vi "TestPanel.vi"() -> ()   [LabVIEW 2018]
uses:
  <vilib>/DAQmx/read.llb/DAQmx Read (Analog 1D Wfm NChan NSamp).vi
  <vilib>/DAQmx/create/channels.llb/DAQmx Create Channel (AI-Voltage-Basic).vi
  <vilib>/DAQmx/configure/timing.llb/DAQmx Timing (Sample Clock).vi
  <vilib>/DAQmx/miscellaneous.llb/DAQmx Fill In Error Info.vi
  <vilib>/measure/madcrms.llb/Basic Averaged DC-RMS for N Chan.vi
  <vilib>/measure/NI_MAPro.lvlib
panel:
  out "Voltage Chart":waveform(dbl)[](graph)
  out "Table Control":string[][](table)
  in  "Stop":bool
  in  "Manual Zero":bool
  # "Test Panel v1.0"
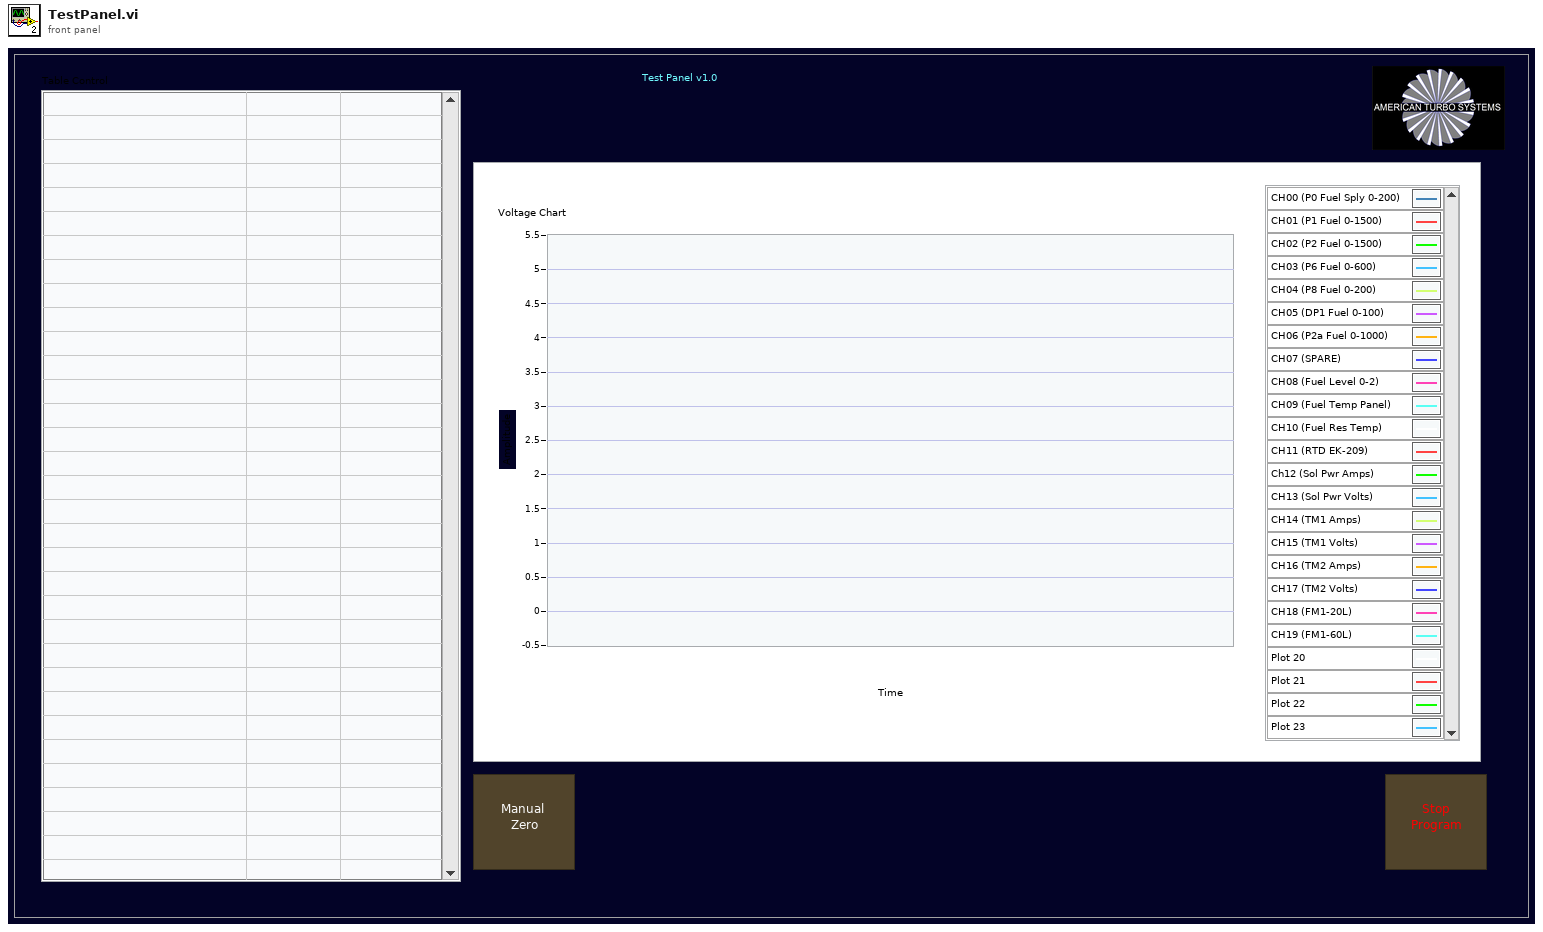
[diagram p1: front panel]
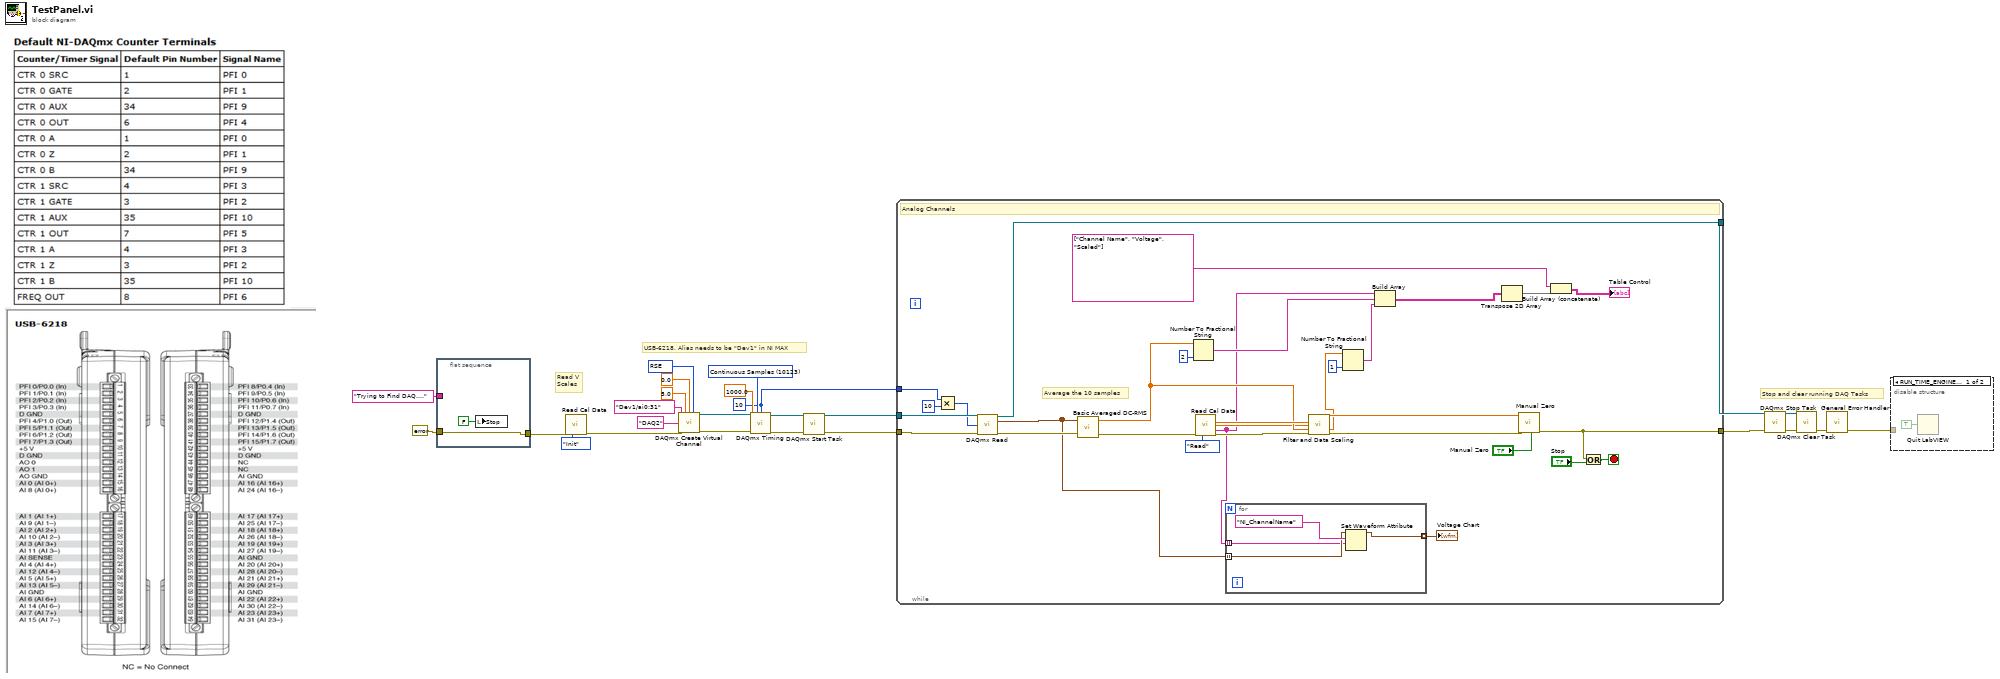
[diagram p0: block diagram]
diagram:
  w4 = 10 ("samples per channel")
  w21 = 10123 items=["Finite Samples"=10178, "Continuous Samples"=10123, "Hardware Timed Single Point"=12522] ("sample mode")
  w18 = 10083 items=["Default"=-1, "RSE"=10083, "NRSE"=10078, "Differential"=10106, "Pseudodifferential"=12529] ("input terminal configuration")
  # "USB-6218. Alias needs to be \"Dev1\" in NI MAX"
  # "Read V\nScales"
  # "Stop and clear running DAQ Tasks"
  n1 = flat-sequence {
    tunnel: errorcluster {"status"=FALSE, "code"=0, "source"=""} ("error in") -> [w26]
    tunnel: [w26] -> w5
    tunnel: "Trying to Find DAQ...." ("ProgramName") -> [_]
    frame #0 {
      n2 = local write "Stop"(FALSE ("stop")) -> ()
    }
  }
  n3 = call "Read Cal Data.vi"("error in (no error)"=w5, "Enum"=enum16{"Init", "Read", "Write"}."Init") -> ("error out"=w1:errorcluster)  [unwired: 1 in, 12 out]
  n4 = call-poly <vilib>:"DAQmx Create Virtual Channel.vi"("maximum value"=5.0, "minimum value"=0.0, "input terminal configuration"=w18, "physical channels"=tag "Dev1/ai0:31", "name to assign"="DAQ2", "error in"=w1) -> ("task out"=w19:refnum<k21>, "error out"=w20:errorcluster)  [unwired: 8 in]
  n5 = call-poly <vilib>:"DAQmx Timing.vi"("task/channels in"=w19, "sample mode"=w21, "samples per channel"=w4, "rate"=1000.0, "error in"=w20) -> ("task out"=w23:refnum<k21>, "error out"=w24:errorcluster)  [unwired: 9 in]
  n6 = call <vilib>:"DAQmx Start Task.vi"("task/channels in"=w23, "error in"=w24) -> ("task out"=w14:refnum<k21>, "error out"=w10:errorcluster)  [unwired: 12 in]
  n7 = while {
    tunnel: w14 -> [w54]
    tunnel: [w53] -> w12
    tunnel: w10 -> [w52]
    tunnel: [w47] -> w8
    tunnel: w4 -> [w44]
    stop <- w46 stop-if-true
    # "Average the 10 samples"
    # "Analog Channels"
    n8 = Multiply(x=w44, y=10) -> (x*y=w45:i32)
    n9 = call-poly <vilib>:"DAQmx Read.vi"("task/channels in"=w54, "number of samples per channel"=w45, "error in"=w52) -> ("task out"=w53:refnum<k21>, "data"=w30:waveform(dbl)[], "error out"=w48:errorcluster)  [unwired: 10 in]
    n10 = call-poly <vilib>:"Basic Averaged DC-RMS.vi"("signals in"=w30) -> ("DC values"=w37:dbl[])  [unwired: 7 in, 3 out]
    n11 = Number To Fractional String(number=w37, precision (6)=i16 2) -> (F-format string=w36:string[])  [unwired: 2 in]
    n12 = call "Read Cal Data.vi"("error in (no error)"=w48, "Enum"=enum16{"Init", "Read", "Write"}."Read") -> ("Slope"=w49:dbl[], "Offset"=w31:dbl[], "Channel Names"=w29:string[], "error out"=w51:errorcluster)  [unwired: 1 in, 9 out]
    n13 = for {
      tunnel: w30 -> [w60] mode=indexing
      tunnel: w29 -> [w59] mode=indexing
      tunnel: [w58] -> w28 mode=indexing
      n14 = Set Waveform Attribute(5:w59, 6:"NI_ChannelName" ("name"), 7:w60) -> (3:w58:waveform(dbl))  [unwired: 1 in, 2 out]
    }
    "Voltage Chart" <- w28
    n15 = call "Filter and Data Scaling.vi"("Slope"=w49, "Offset"=w31, "Vin"=w37, "error in"=w51) -> ("Vout"=w42:dbl[], "ScaledOut"=w34:dbl[], "error out"=w50:errorcluster)  [unwired: 9 in]
    n16 = Number To Fractional String(number=w34, precision (6)=i16 1) -> (F-format string=w35:string[])  [unwired: 2 in]
    n17 = Build Array(w29, w36, w35) -> (w41:string[][])
    n18 = Transpose 2D Array(2D array=w41) -> (transposed array=w40:string[][])
    n19 = call "Manual Zero.vi"("Zero"="Manual Zero", "error in"=w50, "Vin"=w42) -> ("error out"=w47:errorcluster)  [unwired: 2 in, 6 out]
    n20 = Build Array (concatenate)(string[] ["Channel Name", "Voltage", "Scaled"], w40) -> (→"Table Control":string[][])
    n21 = Or(x=w47, y="Stop") -> (x .or. y?=w46:bool)
  }
  n22 = call <vilib>:"DAQmx Stop Task.vi"("task/channels in"=w12, "error in"=w8) -> ("task out"=w13:refnum<k21>, "error out"=w11:errorcluster)  [unwired: 12 in]
  n23 = call <vilib>:"DAQmx Clear Task.vi"("task in"=w13, "error in"=w11) -> ("error out"=w7:errorcluster)  [unwired: 13 in]
  n24 = call <vilib>:"General Error Handler.vi"("error in (no error)"=w7) -> ("error out"=w3:errorcluster)  [unwired: 2 in, 12 out]
  n25 = disable-structure shown="RUN_TIME_ENGINE==True" {
    disable-tunnel: w3 -> [_ _]
    frame condition #0 {
      n26 = Quit LabVIEW(quit? (T)=TRUE) -> ()
    }
    frame condition #1 (active) {
    }
  }
